vi "Read and format refrigerant and mixtures for listbox_d.vi"(6 "error in (no error)":errorcluster, 8 "File names":string[](array[string]), 9 "Refprop Fluid or Mixture Directory":path) -> (0 "error out":errorcluster, 2 "Refrigerant/Mixture Info":string[](array[string]), 3 "Refrigerant/Mixture Name":string[](array[string]))   [LabVIEW 2017]
doc: "Developed by:\nGreg Sussman\nProcess Automation Corp\nwww.processauto.com\n(267)685-1249"
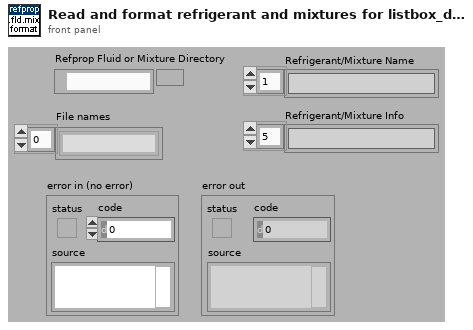
[diagram p1: front panel]
types:
  T1 = enum16{"open", "open or create", "create or replace", "create", "open (read only)"}
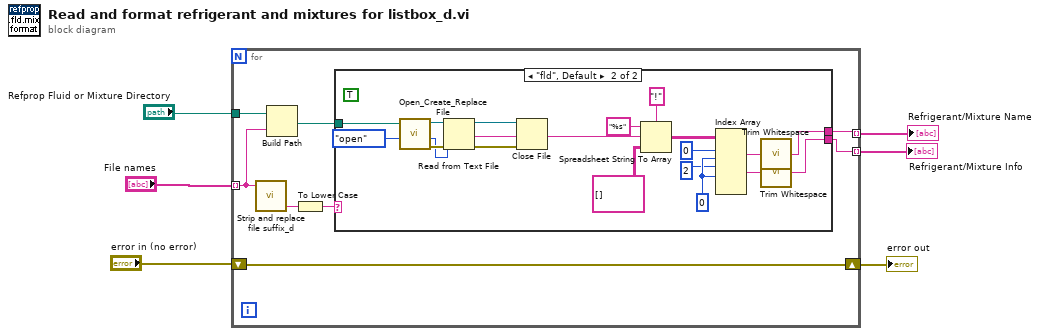
[diagram p0: block diagram]
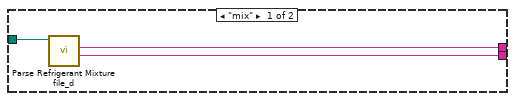
[diagram p2: hidden frame]
diagram:
  n1 = for {
    tunnel: "Refprop Fluid or Mixture Directory" -> [w12]
    tunnel: "File names" -> [w11] mode=indexing
    tunnel: [w9] -> w4 mode=indexing
    tunnel: [w8] -> w3 mode=indexing
    shift-right: [w7] -> w1
    shift-left: "error in (no error)" -> [w7]
    n2 = call "Strip and replace file suffix_d.vi"("File Name"=w11) -> ("Old File Suffix OUT"=w14:string)  [unwired: 3 in, 1 out]
    n3 = Build Path(base path=w12, name or relative path=w11) -> (appended path=w10:path)
    n4 = To Lower Case(string=w14) -> (all lower case string=w13:string)
    n5 = case shown="\"fld\", Default" w13 {
      tunnel: w10 -> [w17 w28]
      tunnel: [w16 w25] -> w9
      tunnel: [w15 w24] -> w8
      frame "mix" {
        n6 = call "Parse Refrigerant Mixture file_d.vi"("Mixture File Path"=w17) -> ("Mixture Definition String"=w15:string, "Mixture Name"=w16:string)  [unwired: 7 in]
      }
      frame "fld", Default {
        (unwired) TRUE ("convert eol (F)")
        w31 = 0 ("disabled index (col)")
        n7 = call <vilib>:"Open_Create_Replace File.vi"("function (open:0)"=T1."open", "file path"=w28) -> ("error out"=w22:errorcluster, "file size (bytes)"=w18:i32, "refnum"=w21:refnum<file>)  [unwired: 6 in, 1 out]
        n8 = Read from Text File(file (use dialog)=w21, count=w18, error in=w22) -> (refnum out=w19:refnum<file>, text=w27:string, error out=w20:errorcluster)  [unwired: 1 in, 1 out]
        n9 = Close File(refnum=w19, error in=w20) -> ()  [unwired: 2 out]
        n10 = Spreadsheet String To Array(delimiter (Tab)="!", format string="%s", spreadsheet string=w27, array type (2D Dbl)=string[][] []) -> (array=w33:string[][])
        n11 = Index Array(array=w33, index (row) #1=0 ("index (row)"), index (col) #1=w31, index (row) #2=2 ("index (row)"), index (col) #2=w31) -> (element #1=w30:string, element #2=w29:string)  [unwired: 2 in, 1 out]
        n12 = call <vilib>:"Trim Whitespace.vi"("string"=w30) -> ("trimmed string"=w25:string)  [unwired: 1 in]
        n13 = call <vilib>:"Trim Whitespace.vi"("string"=w29) -> ("trimmed string"=w24:string)  [unwired: 1 in]
      }
    }
  }
  "Refrigerant/Mixture Name" <- w4
  "Refrigerant/Mixture Info" <- w3
  "error out" <- w1
